vi "iWorx Find myDAQ.vi"(8 "Error In":errorcluster, 10 "Preferred myDAQ (myDAQ1)":tag) -> (0 "Error Out":errorcluster, 1 "myDAQ Found?":bool, 2 "DAQmx Physical Channel":tag, 5 "myDAQs Found":tag[](array[tag]), 7 "# myDAQs Found":i32)   [LabVIEW 2012]
doc: "Locate all connected myDAQ device. Select any myDAQ physical Channel using the <b> Preferred Channel(s) </b> input. If the preferred device is available it will return the correct channel name, if not it will connect to the same channels on the first available myDAQ."
uses:
  <resource>/objmgr/daqmx.rc
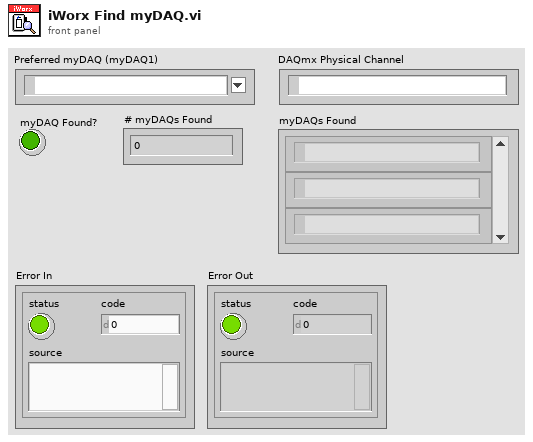
[diagram p1: front panel]
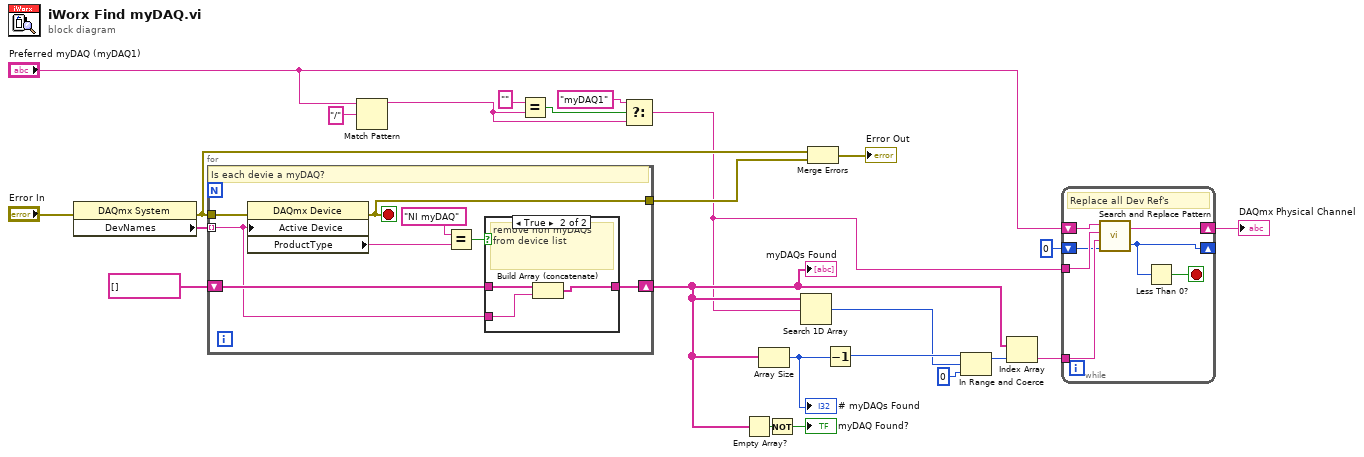
[diagram p0: block diagram]
diagram:
  n1 = property class="DAQmx System"(error in="Error In") -> (error out=w17:errorcluster, "DevNames"=w23:tag[])  [unwired: 1 in, 1 out]
  n2 = for {
    tunnel: w23 -> [w25] mode=indexing
    tunnel: w17 -> [w31]
    tunnel: [w30] -> w16
    shift-right: [w26] -> w14
    shift-left: tag[] [] ("DevNames") -> [w29]
    stop <- w30 stop-if-true
    # "Is each devie a myDAQ?"
    n3 = property class="DAQmx Device"(error in=w31, "Active Device"=w25) -> (error out=w30:errorcluster, "ProductType"=w27:string)  [unwired: 1 in, 1 out]
    n4 = Equal?(x="NI myDAQ" ("y"), y=w27) -> (x = y?=w28:bool)
    n5 = case shown="True" w28 {
      tunnel: w29 -> [w33 w36]
      tunnel: [w33 w34] -> w26
      tunnel: w25 -> [_ w35]
      frame False {
        # "myDAQ detected"
      }
      frame True {
        # "remove non myDAQs from device list"
        n6 = Build Array (concatenate)(w36, w35) -> (w34:tag[])
      }
    }
  }
  "myDAQs Found" <- w14
  n7 = Match Pattern(string="Preferred myDAQ (myDAQ1)", regular expression="/") -> (before substring=w11:string)  [unwired: 1 in, 3 out]
  n8 = Equal?(x="", y=w11) -> (x = y?=w8:bool)
  n9 = Select(t="myDAQ1", s=w8, f=w11) -> (s? t:f=w4:string)
  n10 = Empty Array?(array=w14) -> (empty?=w13:bool)
  n11 = Array Size(array=w14) -> (size(s)=w20:i32)
  "# myDAQs Found" <- w20
  n12 = Not(x=w13) -> (.not. x?=→"myDAQ Found?":bool)
  n13 = Search 1D Array(1D array=w14, element=w4) -> (index of element=w19:i32)  [unwired: 1 in]
  n14 = Merge Errors(w17, w16) -> (→"Error Out":errorcluster)
  n15 = Decrement(x=w20) -> (x-1=w22:i32)
  n16 = In Range and Coerce(upper limit=w22, x=w19, lower limit=0) -> (coerced(x)=w18:i32)  [unwired: 1 out]
  n17 = Index Array(array=w14, index=w18) -> (element=w3:tag)
  n18 = while {
    tunnel: w4 -> [w42]
    tunnel: w3 -> [w40]
    shift-right: [w38] -> _
    shift-left: 0 ("offset past match") -> [w39]
    shift-right: [w41] -> w2
    shift-left: "Preferred myDAQ (myDAQ1)" -> [w43]
    stop <- w37 stop-if-true
    # "Replace all Dev Ref's"
    n19 = call <vilib>:"Search and Replace Pattern.vi"("string"=w43, "regular expression (\"\")"=w42, "replace string (\"\")"=w40, "offset (0)"=w39) -> ("result string"=w41:string, "offset past match"=w38:i32)  [unwired: 1 in]
    n20 = Less Than 0?(x=w38) -> (x < 0?=w37:bool)
  }
  "DAQmx Physical Channel" <- w2
